vi "test_saveMetaData.vi"() -> ()   [LabVIEW 2017]
uses:
  z-axis-params.ctl
  controls/expMetaData.ctl
  <userlib>/_matio/level5/Public/Write/Append Data Element.llb/Append Data Element (Anything).vi
  <userlib>/_matio/level5.lvlib
panel:
  in  "ExpMetaData 2":T1={"xy_error_threshold"=0.1, "xy_settled_samples_threshold"=200, "Ki_xy"=0.005, "state_counts"=[], "TOL"=0.3, "ramp_rate"=-5e-06, "z_u_max"=5.0, "setpoint"=0.0, "Ki"=0.001, "Z_error_threshold"=0.0, "Z_settled_samples_threshold "=0, "z_UP"=1.5, "zup_N"=5000} {"Z_error_threshold" format="%#_13g"; "ramp_rate" format="%#_4g"; "TOL" format="%#_13g"}
  in  "outputData":path
  in  "Array":u64[](array[numeric])
  out "result string":string
  in  "z-axis-params":T2={"TOL"=0.3, "ramp_rate"=-5e-05, "z_u_max"=5.0, "setpoint"=0.0, "Ki"=0.01, "Z_error_threshold"=0.2, "Z_settled_samples_threshold "=500, "z_UP"=1.5, "zup_N"=500} {"Z_error_threshold" format="%#_13g"; "ramp_rate" format="%#_4g"; "TOL" format="%#_13g"}
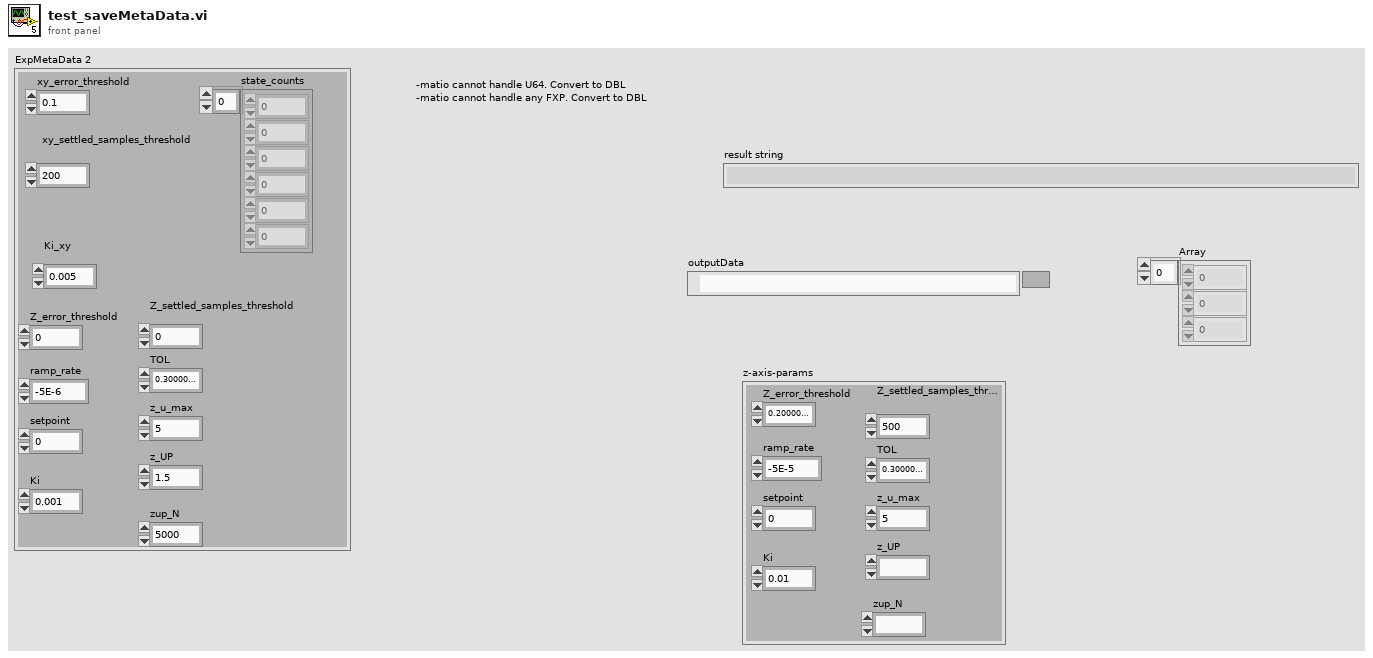
[diagram p1: front panel]
types:
  T1 = typedef "expMetaData.ctl" = cluster{"xy_error_threshold":sgl, "xy_settled_samples_threshold":i16, "Ki_xy":sgl, "state_counts":dbl[], "TOL":sgl, "ramp_rate":sgl, "z_u_max":sgl, "setpoint":sgl, "Ki":sgl, "Z_error_threshold":sgl, "Z_settled_samples_threshold ":i16, "z_UP":sgl, "zup_N":i16}
  T2 = typedef "z-axis-params.ctl" = cluster{"TOL":sgl, "ramp_rate":sgl, "z_u_max":sgl, "setpoint":sgl, "Ki":sgl, "Z_error_threshold":sgl, "Z_settled_samples_threshold ":i16, "z_UP":fxp<+/-,16,5>, "zup_N":i16}
  T3 = enum16{"open", "replace", "create", "open or create", "replace or create", "replace or create with confirmation"}
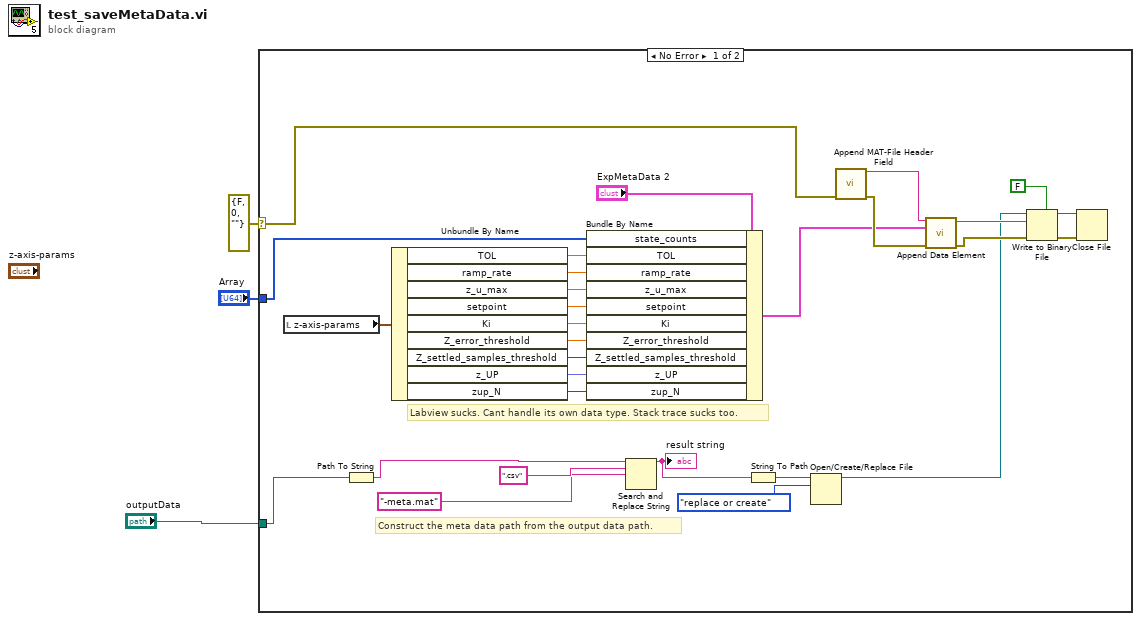
[diagram p0: block diagram]
diagram:
  n1 = case shown="No Error" errorcluster {"status"=FALSE, "code"=0, "source"=""} ("error IO") {
    selector: errorcluster {"status"=FALSE, "code"=0, "source"=""} ("error IO") -> [w21 _]
    tunnel: "outputData" -> [w17 _]
    tunnel: "Array" -> [w4 _]
    frame No Error {
      # "Construct the meta data path from the output data path."
      # "Labview sucks. Cant handle its own data type. Stack trace sucks too."
      n2 = local read "z-axis-params"() -> (w18:T2)
      n3 = Path To String(path=w17) -> (string=w24:string)
      n4 = Unbundle By Name(w18) -> ("TOL"=w14:sgl, "ramp_rate"=w6:sgl, "z_u_max"=w7:sgl, "setpoint"=w8:sgl, "Ki"=w9:sgl, "Z_error_threshold"=w10:sgl, "Z_settled_samples_threshold"=w11:i16, "z_UP"=w12:fxp<+/-,16,5>, "zup_N"=w13:i16)
      n5 = Bundle By Name(cluster="ExpMetaData 2", "state_counts"=w4, "TOL"=w14, "ramp_rate"=w6, "z_u_max"=w7, "setpoint"=w8, "Ki"=w9, "Z_error_threshold"=w10, "Z_settled_samples_threshold"=w11, "z_UP"=w12, "zup_N"=w13) -> (w5:T1)
      n6 = Search and Replace String(input string=w24, search string=".csv", replace string="-meta.mat" ("replace string (\"\")")) -> (result string=w23:string)  [unwired: 5 in, 3 out]
      "result string" <- w23
      n7 = String To Path(string=w23) -> (path=w20:path)
      n8 = Open/Create/Replace File(file path (use dialog)=w20, operation (0:open)=T3."replace or create") -> (refnum out=w19:refnum<file>)  [unwired: 4 in, 2 out]
      n9 = call <userlib>:"Append MAT-File Header Field.vi"("error"=w21) -> ("result string"=w32:string, "error out"=w22:errorcluster)  [unwired: 13 in]
      n10 = call-poly <userlib>:"Append Data Element.vi"("initial string"=w32, "data"=w5, "error in (no error)"=w22) -> ("result string"=w30:string, "error out"=w31:errorcluster)  [unwired: 11 in]
      n11 = Write to Binary File(file (use dialog)=w19, data=w30, error in=w31, 5:FALSE ("prepend array or string size? (T)")) -> (refnum out=w27:refnum<file>, error out=w28:errorcluster)  [unwired: 2 in, 1 out]
      n12 = Close File(refnum=w27, error in=w28) -> ()  [unwired: 2 out]
    }
    frame Error {
    }
  }
